vi "Demo_forces.vi"() -> ()   [LabVIEW 2018]
panel:
  in  "Fz":dbl[](array[numeric])=[0.16, -0.16, 0.19, -0.16, 0.22, -0.16, 0.25, -0.16, 0.28, -0.16, 0.31]
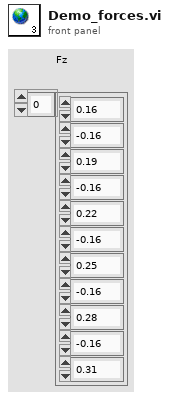
[diagram p1: front panel]
diagram:
